vi "plot_merge_same_filenames.vi"(10 "Input Array":string[][](array[string])=[["a", "a", "b", "a", "d"], ["yep1", "yep2", "nope1", "yep3", "nope2"]]) -> (2 "Output Array":cluster{"1D array":string[][]}[](array[cluster]))   [LabVIEW 2019]
uses:
  ee9c42ca-0c55-3fea-e46a-20ded5b5dd3f.vi
  <vilib>/Array/Sort 2D Array - Pop Stack.vi
  <vilib>/Array/Sort 2D Array - Push Stack.vi
panel:
  # "*******************************************************************\nBiogas Plant Control\n\nAuthor: Paul Zügel\nGCSC-Frankfurt am Main 2020\n\n*******************************************************************"
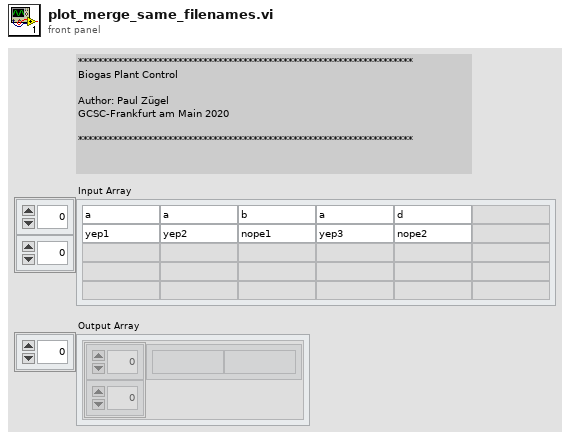
[diagram p1: front panel]
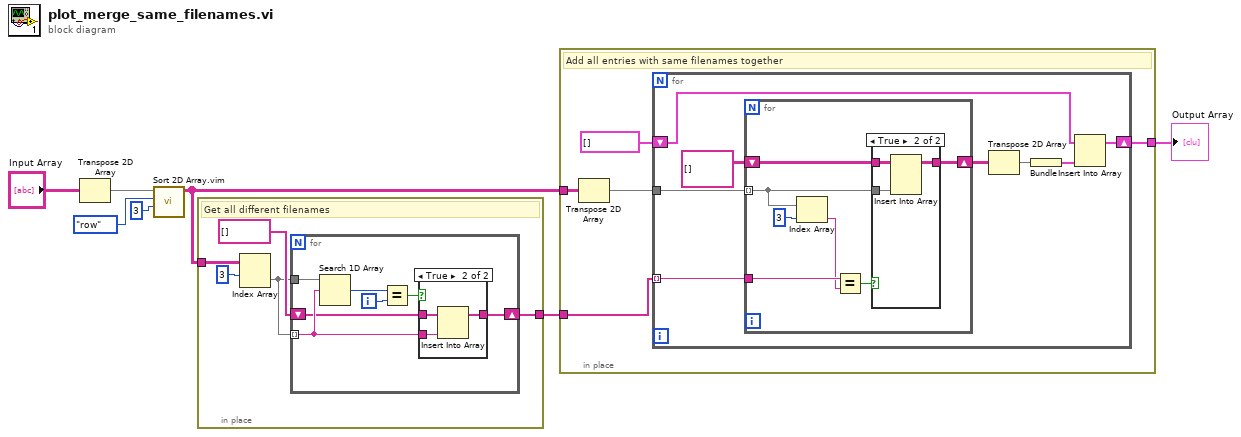
[diagram p0: block diagram]
diagram:
  n1 = Transpose 2D Array(2D array="Input Array") -> (transposed array=w2:string[][])
  n2 = call "Sort 2D Array.vim"("index"=3, "dimension to index (column)"=enum16{"column", "row"}."row", "2D array"=w2) -> ("sorted 2D array"=w4:string[][])  [unwired: 7 in, 1 out]
  n3 = in-place {
    in-place-border: [w9] -> w5
    in-place-border: w4 -> [w8]
    # "Get all different filenames"
    n4 = Index Array(array=w8, index (row)=3) -> (element=w10:string[])  [unwired: 1 in]
    n5 = for {
      shift-right: [w13] -> w9
      shift-left: string[] [] ("1D array") -> [w14]
      tunnel: w10 -> [w16] mode=indexing
      tunnel: w10 -> [w15]
      i -> [w18]
      n6 = Search 1D Array(1D array=w15, element=w16) -> (index of element=w19:i32)  [unwired: 1 in]
      n7 = Equal?(x=w19, y=w18) -> (x = y?=w17:bool)
      n8 = case shown="True" w17 {
        tunnel: w16 -> [_ w22]
        tunnel: w14 -> [w20 w23]
        tunnel: [w20 w21] -> w13
        frame False {
        }
        frame True {
          n9 = Insert Into Array(array=w23, new element=w22) -> (w21:string[])  [unwired: 1 in]
        }
      }
    }
  }
  n10 = in-place {
    in-place-border: w5 -> [w28]
    in-place-border: w4 -> [w26]
    in-place-border: [w25] -> w3
    # "Add all entries with same filenames together"
    n11 = Transpose 2D Array(2D array=w26) -> (transposed array=w27:string[][])
    n12 = for {
      tunnel: w28 -> [w35] mode=indexing
      tunnel: w27 -> [w36]
      shift-right: [w31] -> w25
      shift-left: cluster{"1D array":string[][]}[] [] -> [w32]
      n13 = for {
        tunnel: w36 -> [w37] mode=indexing
        tunnel: w35 -> [w42]
        shift-right: [w39] -> w33
        shift-left: string[][] [] ("1D array") -> [w40]
        n14 = Index Array(array=w37, index=3) -> (element=w38:string)
        n15 = Equal?(x=w42, y=w38) -> (x = y?=w41:bool)
        n16 = case shown="True" w41 {
          tunnel: [w44 w46] -> w39
          tunnel: w40 -> [w44 w47]
          tunnel: w37 -> [_ w45]
          frame False {
          }
          frame True {
            n17 = Insert Into Array(array=w47, new element=w45) -> (w46:string[][])  [unwired: 2 in]
          }
        }
      }
      n18 = Transpose 2D Array(2D array=w33) -> (transposed array=w30:string[][])
      n19 = Bundle(w30) -> (w29:cluster{string[][]})  [unwired: 1 in]
      n20 = Insert Into Array(array=w32, new element=w29) -> (w31:cluster{"1D array":string[][]}[])  [unwired: 1 in]
    }
  }
  "Output Array" <- w3
